vi "PostUserInterfaceRefnum.vi"(8 "error in (no error)":errorcluster, 9 "VI Refnum":refnum<vi>, 10 "Panel":string, 11 "DataProcessor in":refnum<class "DataProcessor.lvclass">) -> (0 "error out":errorcluster, 3 "DataProcessor out":refnum<class "DataProcessor.lvclass">)   [LabVIEW 2020, in "DataProcessor.lvlib" / "DataProcessor.lvclass"]
uses:
  DataProcessor.lvclass
  C:/Program Files/National Instruments/LabVIEW 2020/vi.lib/ActorFramework/Actor/Actor.lvclass
  <vilib>/ActorFramework/Actor/Actor.lvclass/Actor.ctl
  Interface/DockStation Messages/InsertDevicePanel Msg/InsertDevicePanel Msg.lvclass/InsertDevicePanel Msg.ctl
  <vilib>/ActorFramework/Message Enqueuer/Message Enqueuer.lvclass/Message Enqueuer.ctl
  <vilib>/ActorFramework/Message Enqueuer/Enqueue.vi
  Interface/DockStation Messages/InsertDevicePanel Msg/InsertDevicePanel Msg.lvclass
  C:/Program Files/National Instruments/LabVIEW 2020/vi.lib/ActorFramework/Message/Message.lvclass
  <vilib>/ActorFramework/Message Priority Queue/Priority Enqueue.vi
  <vilib>/ActorFramework/Actor/Actor.lvclass
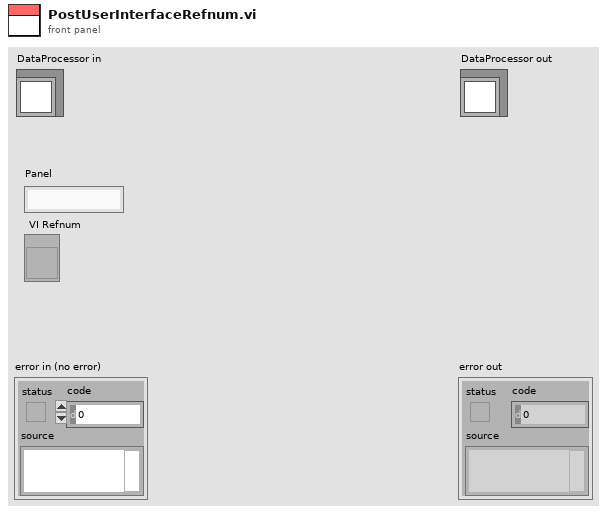
[diagram p1: front panel]
types:
  T1 = enum32{"Invalid", "Standard", "Closed", "Hidden", "Minimized", "Maximized"}
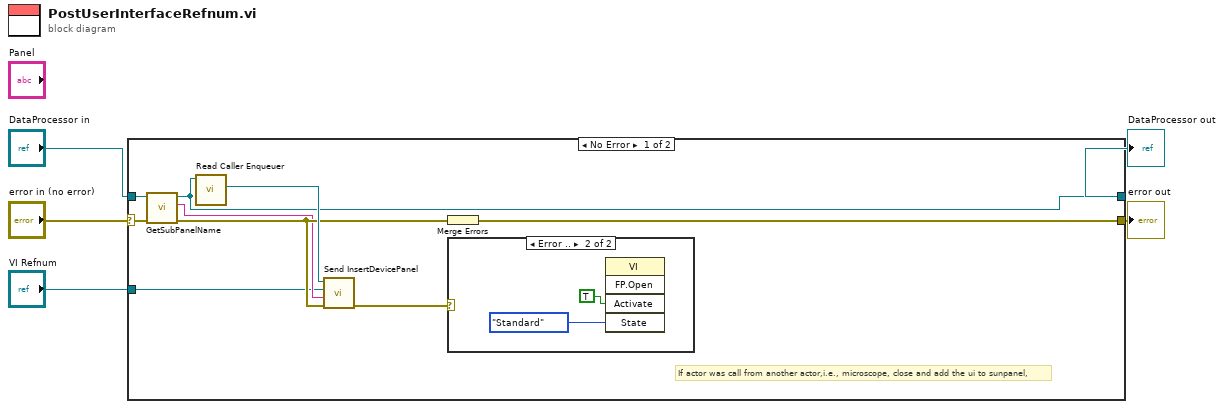
[diagram p0: block diagram]
diagram:
  n1 = case shown="No Error" "error in (no error)" {
    selector: "error in (no error)" -> [w11 w18]
    tunnel: [w14 w18] -> w4
    tunnel: [w8 w17] -> w5
    tunnel: "DataProcessor in" -> [w9 w17]
    tunnel: "VI Refnum" -> [w6 _]
    frame No Error {
      # "If actor was call from another actor,i.e., microscope, close and add the ui to sunpanel,"
      n2 = call-dynamic "GetSubPanelName.vi"("error in (no error)"=w11, "DataProcessor in"=w9) -> ("error out"=w10:errorcluster, "Panel"=w7:string, "DataProcessor out"=w8:refnum<class "DataProcessor.lvclass">)  [unwired: 7 in]
      n3 = call <vilib>:"Read Caller Enqueuer.vi"("Actor"=w8) -> ("Caller Enqueuer"=w13:refnum<class "Message Enqueuer.lvclass">)  [unwired: 10 in]
      n4 = call "Send InsertDevicePanel.vi"("error in (no error)"=w10, "Panel"=w7, "VI Refnum"=w6, "Message Enqueuer"=w13) -> ("error out"=w12:errorcluster)  [unwired: 6 in, 1 out]
      n5 = Merge Errors(w10) -> (w14:errorcluster)
      n6 = case shown="Error .." w12 {
        frame No Error {
        }
        frame Error {
          n7 = invoke class="VI" method="FP.Open"("Activate"=TRUE ("Activate?"), "State"=T1."Standard") -> ()  [unwired: 3 in, 5 out]
        }
      }
    }
    frame Error {
    }
  }
  "error out" <- w4
  "DataProcessor out" <- w5
